vi "Draw.vi"(8 "error in (no error)":errorcluster, 9 "disable contained items?":bool, 10 "IB_SourceTree in":refnum<class "IB_Tree.lvclass">, 11 "IB_TreeBuildSpecs in":refnum<class "IB_Tree_Item_Proj_BuildSpecs.lvclass">) -> (0 "error out":errorcluster, 3 "IB_TreeRootItem out":refnum<class "IB_Tree_Item_Proj_BuildSpecs.lvclass">)   [LabVIEW 2020, in "IB_Tree_Item_Proj_BuildSpecs.lvclass"]
uses:
  <vilib>/AppBuilder/IB_Classes/Tree_Item_Proj_BuildSpecs/IB_Tree_Item_Proj_BuildSpecs.lvclass
  <vilib>/AppBuilder/IB_Classes/Tree_Item_Proj_BuildSpecs/IB_Tree_Item_Proj_BuildSpecs.lvclass/IB_Tree_Item_Proj_BuildSpecs.ctl
  <resource>/Framework/Providers/Builds/Installer/controls/IB_Tree_DefaultSymbols.ctl
  <vilib>/AppBuilder/IB_Classes/Tree_Source/IB_Tree_Source.lvclass
  <vilib>/AppBuilder/IB_Classes/Tree/IB_Tree.lvclass
  <vilib>/AppBuilder/IB_Classes/Tree_Item/IB_Tree_Item.lvclass
  <vilib>/AppBuilder/IB_Classes/Tree_Item_Proj/IB_Tree_Item_Proj.lvclass
  e:/builds/penguin/labview/branches/2020/dev/dist/vi.lib/AppBuilder/IB_Classes/Tree_Item_Proj_Container/IB_Tree_Item_Proj_Container.lvclass
  e:/builds/penguin/labview/branches/2020/dev/dist/vi.lib/AppBuilder/IB_Classes/Tree_Item_Proj/IB_Tree_Item_Proj.lvclass
  e:/builds/penguin/labview/branches/2020/dev/dist/vi.lib/AppBuilder/IB_Classes/Tree_Item/IB_Tree_Item.lvclass
  e:/builds/penguin/labview/branches/2020/dev/dist/vi.lib/AppBuilder/IB_Classes/Tree_Item_Proj_BuildSpecs/IB_Tree_Item_Proj_BuildSpecs.lvclass
  e:/builds/penguin/labview/branches/2020/dev/dist/vi.lib/AppBuilder/IB_Classes/Tree/IB_Tree.lvclass
  e:/builds/penguin/labview/branches/2020/dev/dist/vi.lib/AppBuilder/IB_Classes/Tree_Source/IB_Tree_Source.lvclass
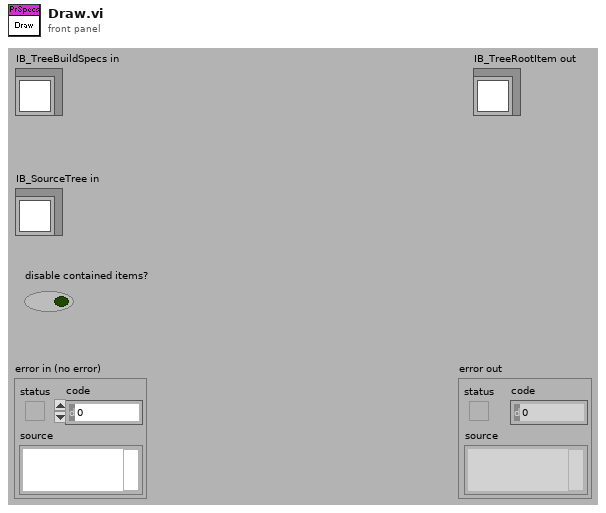
[diagram p1: front panel]
types:
  T1 = typedef "IB_Tree_DefaultSymbols.ctl" = enum16{"<unknown>", "closed folder", "open folder", "closed folder (default)", "open folder (default)", "closed sync folder", "open sync folder", "container folder", "my computer", "build specs", "exe", "dll", "source dist", "restful web service", ".net", "packed library", "c-generator", "target"}
  T2 = typedef "IB_Tree_Source.ctl" = cluster{"buildObject":T3}
  T3 = typedef "ItemRef.ctl" = u64
  T4 = typedef "IB_Tree_Item_Proj.ctl" = cluster{"itemID":string, "path":path}
  T5 = typedef "IB_Tree_Item.ctl" = cluster{"symbol index":i32, "child tag":string, "parentTag":string, "left cell name":string}
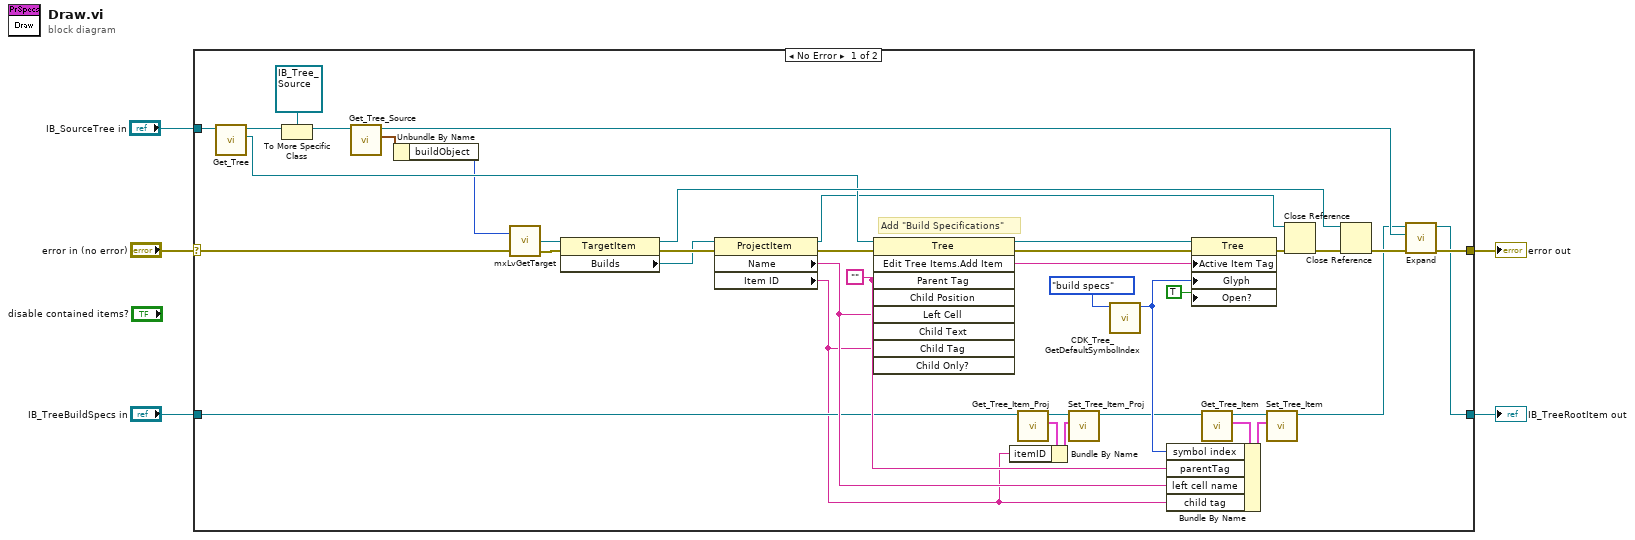
[diagram p0: block diagram]
diagram:
  n1 = case shown="No Error" "error in (no error)" {
    selector: "error in (no error)" -> [w7 w46]
    tunnel: [w21 w46] -> w4
    tunnel: [w10 w45] -> w5
    tunnel: "IB_SourceTree in" -> [w35 _]
    tunnel: "IB_TreeBuildSpecs in" -> [w14 w45]
    frame No Error {
      w26 = ""
      # "Add \"Build Specifications\""
      n2 = call <vilib>:"Get_Tree.vi"("IB_Tree in"=w35) -> ("ctl"=w36:refnum<vi>, "IB_Tree out"=w31:refnum<class "IB_Tree.lvclass">)  [unwired: 1 in, 8 out]
      n3 = To More Specific Class(target class=refnum<class "IB_Tree_Source.lvclass"> refnum ("IB_SourceTree.lvclass"), reference=w31) -> (specific class reference=w30:refnum<class "IB_Tree_Source.lvclass">)  [unwired: 1 in, 1 out]
      n4 = call <vilib>:"Get_Tree_Source.vi"("IB_SourceTree in"=w30) -> ("data"=w37:T2, "IB_SourceTree out"=w20:refnum<class "IB_Tree_Source.lvclass">)  [unwired: 1 in, 8 out]
      n5 = Unbundle By Name(w37) -> ("buildObject"=w9:T3)
      n6 = call <resource>:"mxLvGetTarget.vi"("Item"=w9, "error in"=w7) -> ("Target"=w8:refnum<vi>, "error out"=w6:errorcluster)  [unwired: 1 out]
      n7 = property class="TargetItem"(reference=w8, error in=w6) -> (reference out=w42:refnum<vi>, error out=w44:errorcluster, "Builds"=w38:refnum<vi>)
      n8 = property class="ProjectItem"(reference=w38, error in=w44) -> (reference out=w24:refnum<vi>, error out=w41:errorcluster, "Name"=w25:string, "Item ID"=w12:string)
      n9 = invoke class="Tree" method="Edit Tree Items.Add Item"(reference=w36, error in=w41, "Parent Tag"=w26, "Left Cell"=w25, "Child Tag"=w12) -> (reference out=w39:refnum<vi>, error out=w33:errorcluster, "Edit Tree Items:Add Item"=w11:string)  [unwired: 4 in, 6 out]
      n10 = call <vilib>:"Get_Tree_Item_Proj.vi"("IB_TreeProjectItem in"=w14) -> ("data"=w16:T4, "IB_TreeProjectItem out"=w17:refnum<class "IB_Tree_Item_Proj_BuildSpecs.lvclass">)  [unwired: 1 in, 8 out]
      n11 = Bundle By Name(cluster=w16, "itemID"=w12) -> (w15:T4)
      n12 = call <vilib>:"Set_Tree_Item_Proj.vi"("data"=w15, "IB_TreeProjectItem in"=w17) -> ("IB_TreeProjectItem out"=w13:refnum<class "IB_Tree_Item_Proj_BuildSpecs.lvclass">)  [unwired: 1 in, 8 out]
      n13 = call <resource>:"CDK_Tree_GetDefaultSymbolIndex.vi"("default symbol"=IB_Tree_DefaultSymbols."build specs") -> ("symbol index"=w18:i32)  [unwired: 1 in, 9 out]
      n14 = property class="Tree"(reference=w39, error in=w33, "Active Item Tag"=w11, "Glyph"=w18, "Open?"=TRUE ("Active Item:Open?")) -> (error out=w23:errorcluster)  [unwired: 1 out]
      n15 = call <vilib>:"Get_Tree_Item.vi"("IB_TreeItem in"=w13) -> ("data"=w28:T5, "IB_TreeItem out"=w29:refnum<class "IB_Tree_Item_Proj_BuildSpecs.lvclass">)  [unwired: 1 in, 8 out]
      n16 = Bundle By Name(cluster=w28, "symbol index"=w18, "parentTag"=w26, "left cell name"=w25, "child tag"=w12) -> (w27:T5)
      n17 = call <vilib>:"Set_Tree_Item.vi"("data"=w27, "IB_TreeItem in"=w29) -> ("IB_TreeItem out"=w19:refnum<class "IB_Tree_Item_Proj_BuildSpecs.lvclass">)  [unwired: 1 in, 8 out]
      n18 = Close Reference(reference=w24, error in (no error)=w23) -> (error out=w43:errorcluster)
      n19 = Close Reference(reference=w42, error in (no error)=w43) -> (error out=w22:errorcluster)
      n20 = call-dynamic "Expand.vi"("error in (no error)"=w22, "IB_Tree.lvclass"=w20, "IB_TreeRootItem in"=w19) -> ("error out"=w21:errorcluster, "IB_TreeRootItem out"=w10:refnum<class "IB_Tree_Item_Proj_BuildSpecs.lvclass">)  [unwired: 7 out]
    }
    frame Error {
    }
  }
  "error out" <- w4
  "IB_TreeRootItem out" <- w5
